vi "State machine program.vi"() -> ()   [LabVIEW 2013]
uses:
  <vilib>/DAQmx/read.llb/DAQmx Read (Analog 2D DBL NChan NSamp).vi
  <vilib>/DAQmx/create/channels.llb/DAQmx Create Channel (AI-Voltage-Basic).vi
  <vilib>/DAQmx/configure/timing.llb/DAQmx Timing (Sample Clock).vi
  <vilib>/DAQmx/miscellaneous.llb/DAQmx Fill In Error Info.vi
panel:
  in  "Tare":bool
  out "appended array":dbl[][](array[numeric])
  in  "stop":bool
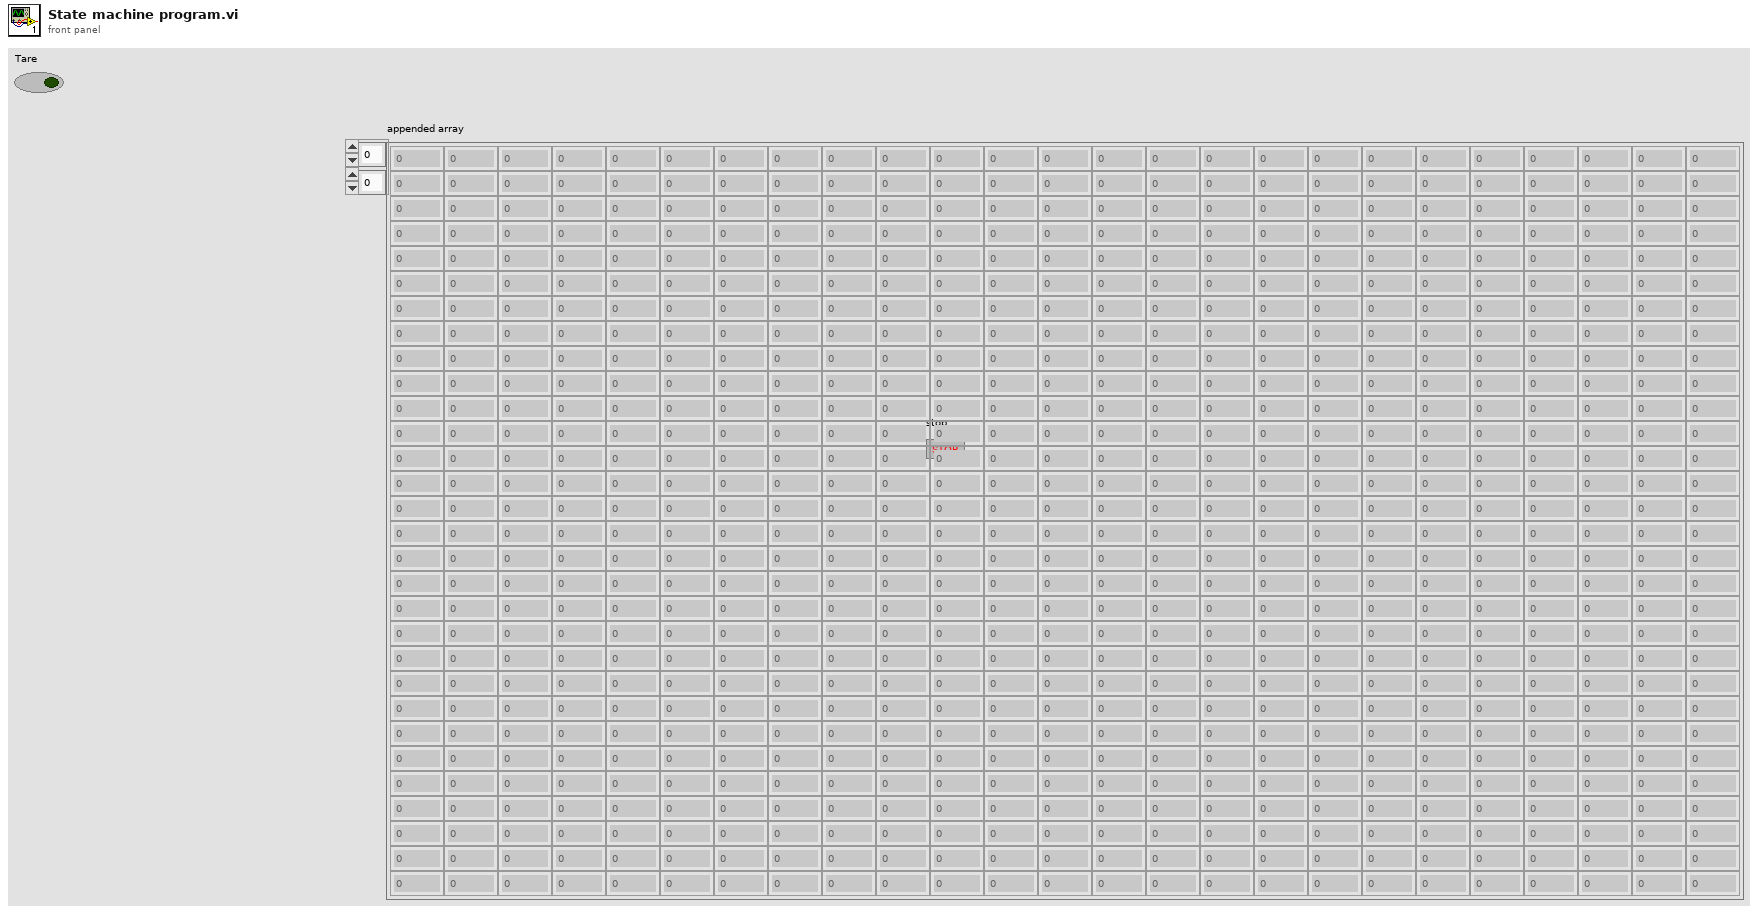
[diagram p1: front panel]
types:
  T1 = enum16{"Initialize", "Setup task", "Setup channel", "Acquire data", "Shutdown task", "Shutdown"}
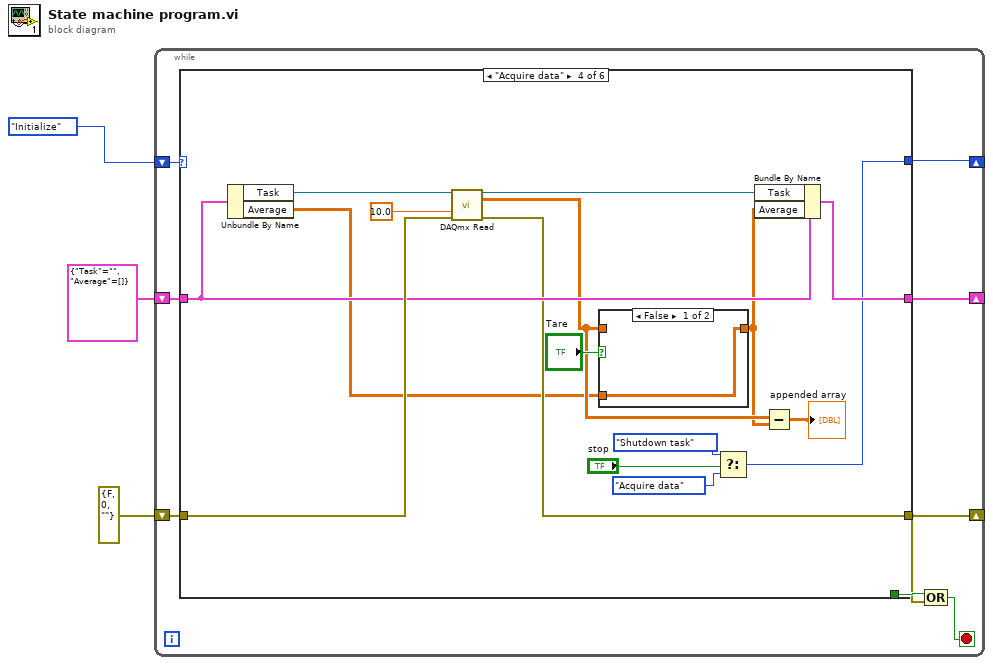
[diagram p0: block diagram]
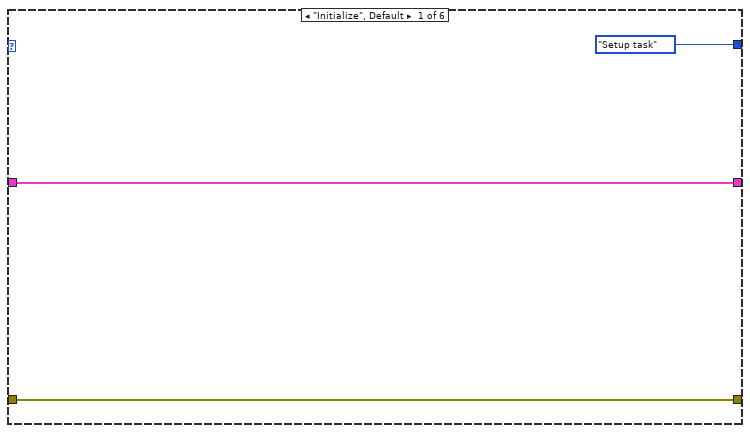
[diagram p2: hidden frame]
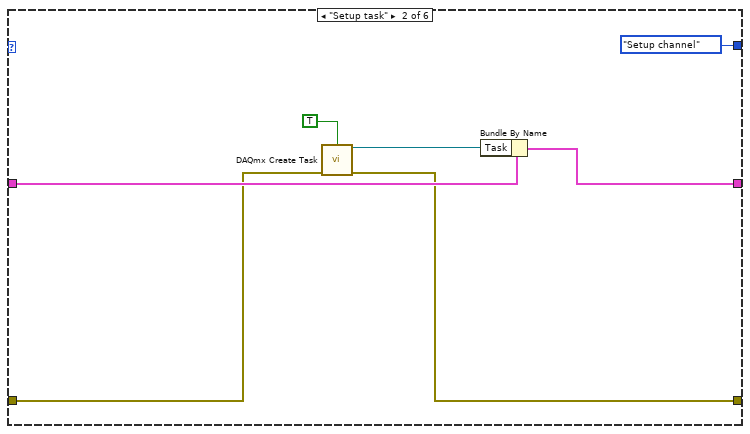
[diagram p3: hidden frame]
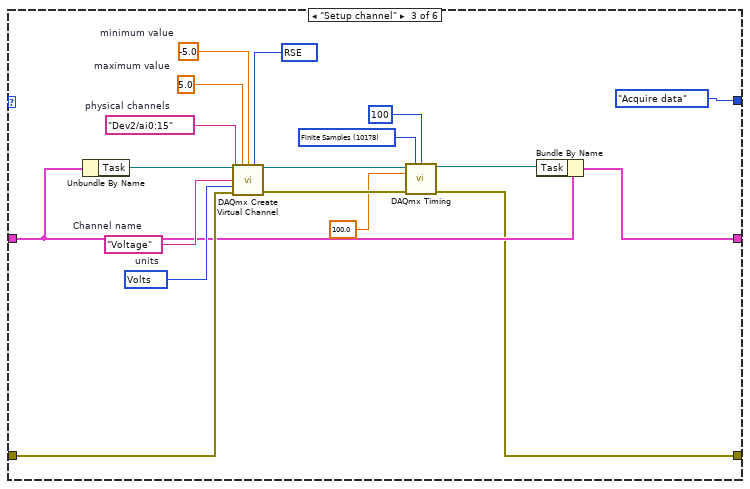
[diagram p4: hidden frame]
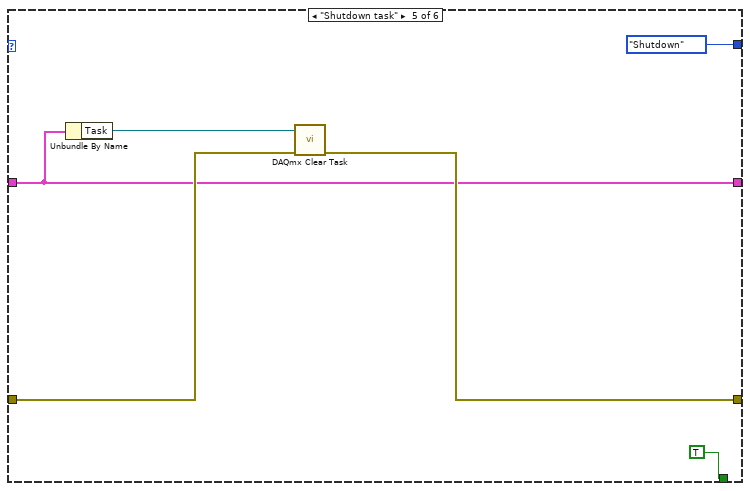
[diagram p6: hidden frame]
diagram:
  n1 = while {
    shift-right: [w4] -> _
    shift-left: errorcluster {"status"=FALSE, "code"=0, "source"=""} ("error in (no error)") -> [w11]
    shift-right: [w7] -> _
    shift-left: T1."Initialize" -> [w10]
    shift-right: [w8] -> _
    shift-left: cluster{"Task":refnum<k21>, "Average":dbl[][]} {"Task"="", "Average"=[]} -> [w9]
    stop <- w5 stop-if-true
    n2 = case shown="\"Acquire data\"" w10 {
      tunnel: w11 -> [w12 w18 w32 w54 w63 w64]
      tunnel: w9 -> [w13 w20 w28 w53 w58 w65]
      tunnel: [w13 w19 w26 w52 w58 w65] -> w8
      tunnel: [T1."Setup task" T1."Setup channel" T1."Acquire data" w47 T1."Shutdown" _] -> w7
      tunnel: [_ _ _ _ TRUE _] -> w6
      tunnel: [w12 w17 w27 w51 w60 w64] -> w4
      frame "Initialize", Default {
      }
      frame "Setup task" {
        n3 = call <vilib>:"DAQmx Create Task.vi"("auto cleanup"=TRUE, "error in"=w18) -> ("task out"=w21:refnum<k21>, "error out"=w17:errorcluster)  [unwired: 12 in]
        n4 = Bundle By Name(cluster=w20, "Task"=w21) -> (w19:cluster{"Task":refnum<k21>, "Average":dbl[][]})
      }
      frame "Setup channel" {
        w25 = 10178 items=["Finite Samples"=10178, "Continuous Samples"=10123, "Hardware Timed Single Point"=12522] ("sample mode")
        w33 = 10348 items=["Volts"=10348, "From Custom Scale"=10065]  # units
        w34 = "Voltage"  # Channel name
        w36 = tag "Dev2/ai0:15"  # physical channels
        w37 = 10083 items=["Default"=-1, "RSE"=10083, "NRSE"=10078, "Differential"=10106, "Pseudodifferential"=12529] ("input terminal configuration")
        w38 = -5.0  # minimum value
        w39 = 5.0  # maximum value
        n5 = Unbundle By Name(w28) -> ("Task"=w35:refnum<k21>)
        n6 = call-poly <vilib>:"DAQmx Create Virtual Channel.vi"("task in"=w35, "maximum value"=w39, "minimum value"=w38, "input terminal configuration"=w37, "physical channels"=w36, "name to assign"=w34, "units"=w33, "error in"=w32) -> ("task out"=w31:refnum<k21>, "error out"=w30:errorcluster)  [unwired: 6 in]
        n7 = call-poly <vilib>:"DAQmx Timing.vi"("task/channels in"=w31, "sample mode"=w25, "samples per channel"=100, "rate"=100.0, "error in"=w30) -> ("task out"=w29:refnum<k21>, "error out"=w27:errorcluster)  [unwired: 9 in]
        n8 = Bundle By Name(cluster=w28, "Task"=w29) -> (w26:cluster{"Task":refnum<k21>, "Average":dbl[][]})
      }
      frame "Acquire data" {
        n9 = Unbundle By Name(w53) -> ("Task"=w55:refnum<k21>, "Average"=w41:dbl[][])
        n10 = call-poly <vilib>:"DAQmx Read.vi"("task/channels in"=w55, "timeout"=10.0, "error in"=w54) -> ("task out"=w45:refnum<k21>, "data"=w43:dbl[][], "error out"=w51:errorcluster)  [unwired: 10 in]
        n11 = case shown="False" "Tare" {
          tunnel: w43 -> [_ w57]
          tunnel: [w56 w57] -> w40
          tunnel: w41 -> [w56 _]
          frame False {
          }
          frame True {
          }
        }
        n12 = Select(t=T1."Shutdown task", s="stop", f=T1."Acquire data") -> (s? t:f=w47:T1)
        n13 = Bundle By Name(cluster=w53, "Task"=w45, "Average"=w40) -> (w52:cluster{"Task":refnum<k21>, "Average":dbl[][]})
        n14 = Subtract(x=w43, y=w40) -> (x-y=→"appended array":dbl[][])
      }
      frame "Shutdown task" {
        n15 = Unbundle By Name(w58) -> ("Task"=w62:refnum<k21>)
        n16 = call <vilib>:"DAQmx Clear Task.vi"("task in"=w62, "error in"=w63) -> ("error out"=w60:errorcluster)  [unwired: 13 in]
      }
      frame "Shutdown" {
      }
    }
    n17 = Compound Arithmetic op=OR(w6, w4) -> (w5:bool)
  }
